vi "CRD HF v3.vi"   [LabVIEW 2017]
uses:
  <vilib>/rvi/eio/nirviErrorMerge/nirviErrorMerge.xnode
  <vilib>/rvi/eio/common/nirviEmuClasses.ctl
  <vilib>/rvi/eio/common/nirviEmuTemplateMethod_errors.vi
  <vilib>/rvi/eio/nirviEIOMethodImplementation/nirviEIOMethodImplementation.xnode
  <vilib>/eio/EIOGrowableMethodNode/genericMethod/EIOGrowableMethodNode.xnode
  <vilib>/rvi/DataTransferAndStorage/Container/XNode/niFpgaContainer.xnode
  <vilib>/rvi/DataTransferAndStorage/Register/Emulation/niFpgaRegisterEmulation.vi
  <vilib>/eio/EIONode/EIONode.xnode
  <vilib>/rvi/FIFO/Fifo_Resource/nirvififoEmulationWrite.vi
  <vilib>/rvi/FIFO/Fifo_Resource/nirvififoEmulationRead.vi
types:
  T1 = typedef "nirviEmuClasses.ctl" = enum16{"IO Read", "IO Write", "Method", "Property Read", "Property Write"}
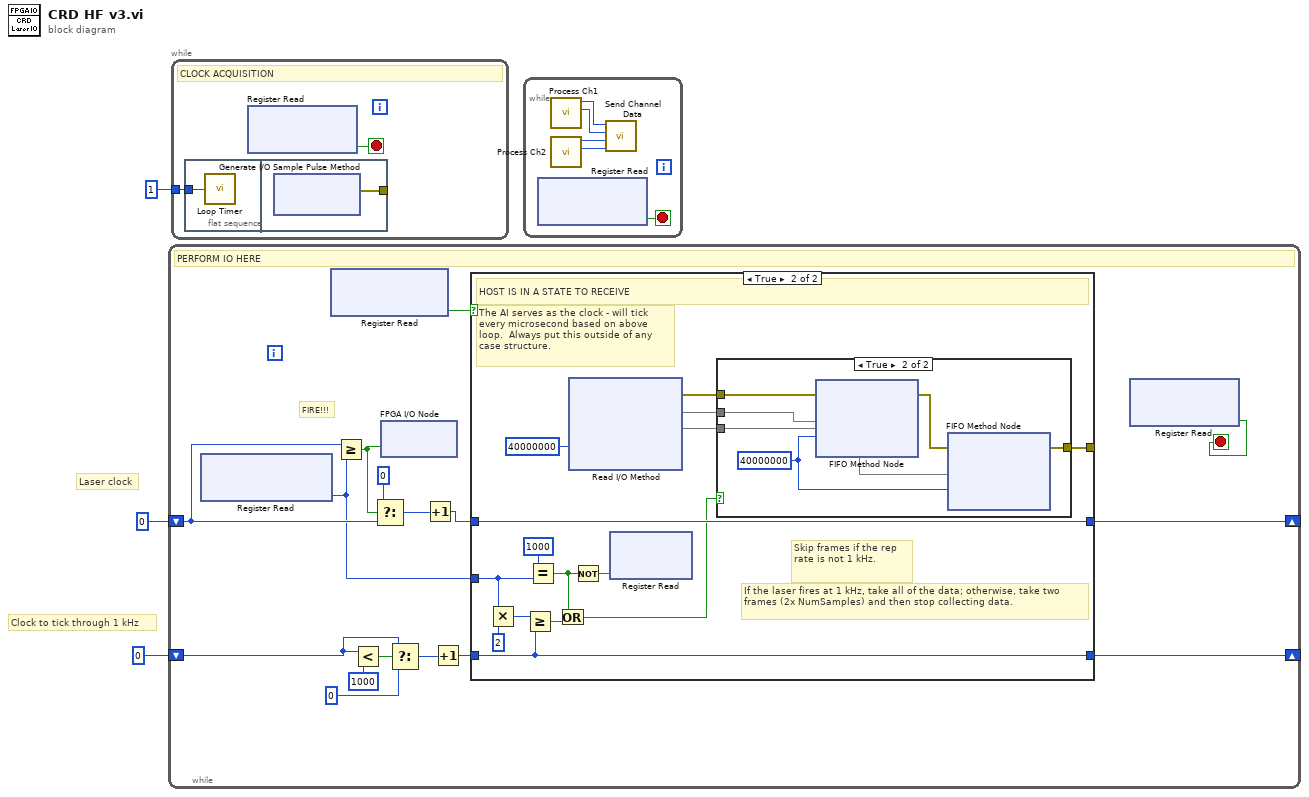
[diagram p0: block diagram]
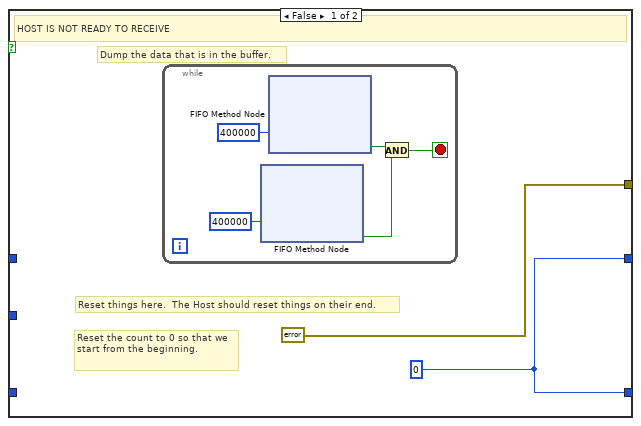
[diagram p2: hidden frame]
diagram:
  # "Laser clock"
  # "Clock to tick through 1 kHz"
  n1 = while {
    shift-right: [w16] -> _
    shift-left: u16 0 ("Number of Samples") -> [w17]
    shift-right: [w7] -> _
    shift-left: u16 0 ("Number of Samples") -> [w5]
    stop <- w4 stop-if-true
    # "FIRE!!!"
    # "PERFORM IO HERE"
    n2 = xnode ("Register Read")() -> ("Data"=w10:u16)  [unwired: 1 in, 1 out]
    n3 = xnode ("Register Read")() -> ("Data"=w13:bool)  [unwired: 1 in, 1 out]
    n4 = Greater Or Equal?(x=w17, y=w10) -> (x >= y?=w18:bool)
    n5 = Less?(x=w5, y=u16 1000) -> (x < y?=w9:bool)
    n6 = Select(t=u16 0 ("Number of Samples"), s=w18, f=w17) -> (s? t:f=w15:u16)
    n7 = xnode "FPGA I/O Node"("CRDS"=w18) -> ()  [unwired: 1 in, 1 out]
    n8 = Select(t=w5, s=w9, f=u16 0 ("Number of Samples")) -> (s? t:f=w12:u16)
    n9 = Increment(x=w15) -> (x+1=w14:u16)
    n10 = Increment(x=w12) -> (x+1=w8:u16)
    n11 = case shown="True" w13 {
      tunnel: [errorcluster {"Status?"=FALSE, "Code"=0, "Source"=""} ("error out") w27] -> _
      tunnel: w14 -> [_ w41]
      tunnel: [w20 w41] -> w16
      tunnel: w10 -> [_ w37]
      tunnel: w8 -> [_ w32]
      tunnel: [w20 w32] -> w7
      frame False {
        w20 = u16 0 ("Number of Samples")
        # "Dump the data that is in the buffer."
        # "Reset things here.  The Host should reset things on their end."
        # "Reset the count to 0 so that we start from the beginning."
        # "HOST IS NOT READY TO RECEIVE"
        n12 = while {
          stop <- w22 stop-if-true
          n13 = xnode ("FIFO Method Node")("Timeout"=400000) -> ("Timed Out?"=w23:bool)  [unwired: 1 in, 2 out]
          n14 = xnode ("FIFO Method Node")("Timeout"=400000) -> ("Timed Out?"=w24:bool)  [unwired: 1 in, 2 out]
          n15 = And(x=w24, y=w23) -> (x .and. y?=w22:bool)
        }
      }
      frame True {
        # "The AI serves as the clock - will tick every microsecond based on above loop.  Always put this outside of any case structure."
        # "Skip frames if the rep rate is not 1 kHz."
        # "If the laser fires at 1 kHz, take all of the data; otherwise, take two frames (2x NumSamples) and then stop collecting data."
        # "HOST IS IN A STATE TO RECEIVE"
        n16 = Multiply(x=w37, y=u16 2) -> (x*y=w35:u16)
        n17 = Greater Or Equal?(x=w35, y=w32) -> (x >= y?=w34:bool)
        n18 = Equal?(x=u16 1000, y=w37) -> (x = y?=w39:bool)
        n19 = Or(x=w39, y=w34) -> (x .or. y?=w33:bool)
        n20 = xnode "Read I/O Method"("Timeout"=40000000) -> ("error out"=w29:errorcluster, "CRD Las Ch 1"=w30, "CRD Las Ch 2"=w28)  [unwired: 1 in, 1 out]
        n21 = Not(x=w39) -> (.not. x?=w38:bool)
        n22 = xnode ("Register Read")("Data"=w38) -> ()  [unwired: 1 in, 1 out]
        n23 = case shown="True" w33 {
          tunnel: w30 -> [_ w156]
          tunnel: w29 -> [w150 w155]
          tunnel: w28 -> [_ w153]
          tunnel: [w150 w151] -> w27
          frame False {
          }
          frame True {
            w154 = 40000000 ("Timeout")
            n24 = xnode ("FIFO Method Node")("Element"=w156, "Timeout"=w154, "error in (no error)"=w155) -> ("error out"=w152:errorcluster)  [unwired: 1 in, 2 out]
            n25 = xnode ("FIFO Method Node")("Element"=w153, "Timeout"=w154, "error in (no error)"=w152) -> ("error out"=w151:errorcluster)  [unwired: 1 in, 2 out]
          }
        }
      }
    }
    n26 = xnode ("Register Read")() -> ("Data"=w4:bool)  [unwired: 1 in, 1 out]
  }
  n27 = while {
    tunnel: u32 1 ("Sample Period (uSec)") -> [w158]
    stop <- w157 stop-if-true
    # "CLOCK ACQUISITION"
    n28 = flat-sequence {
      tunnel: w158 -> [w159]
      tunnel: [w160] -> _
      frame #0 {
        n29 = call "Loop Timer"("Count(uSec)"=w159) -> ()  [unwired: 1 out]
      }
      frame #1 {
        n30 = xnode "Generate I/O Sample Pulse Method"() -> ("error out"=w160:errorcluster)  [unwired: 1 in]
      }
    }
    n31 = xnode ("Register Read")() -> ("Data"=w157:bool)  [unwired: 1 in, 1 out]
  }
  n32 = while {
    stop <- w209 stop-if-true
    n33 = xnode ("Register Read")() -> ("Data"=w209:bool)  [unwired: 1 in, 1 out]
    n34 = call "Process Ch1.vi"() -> ("Max1"=w207:u32, "Max0"=w208:u32)  [unwired: 10 in]
    n35 = call "Process Ch2.vi"() -> ("Max4"=w205:u32, "Max3"=w206:u32)  [unwired: 10 in]
    n36 = call "Send Channel Data.vi"("Max3"=w205, "Max2"=w206, "Max1"=w207, "Max0"=w208) -> ()  [unwired: 8 in]
  }
